vi "Start.vi"(8 "error in (no error)":errorcluster, 10 "Message in":refnum<class "StartMessage.lvclass">, 11 "wavefront sensor in":refnum<class "wavefront sensor.lvclass">) -> (0 "error out":errorcluster, 3 "wavefront sensor out":refnum<class "wavefront sensor.lvclass">)   [LabVIEW 2012, in "wavefront sensor.lvclass"]
doc: "This member function is called when the statemachine in the run.vi receives an 'start' command. It relays the message to all observers of the component.\n\nOverride this member function in your derived class if you need additional start functionality (but don't forget to call the parent method)."
uses:
  wavefront sensor.lvclass
  <vilib>/Distrio/Murmex/StartMessage/StartMessage.lvclass
  <vilib>/Distrio/Murmex/Murmex/Murmex.lvclass
panel:
  # "This member function is called when the statemachine in the run.vi receives an 'start' command. It relays the message to all observers of the component.\n\nOverride this member function in your derived class if you need additional start functionality (but don't forget to call the parent method)."
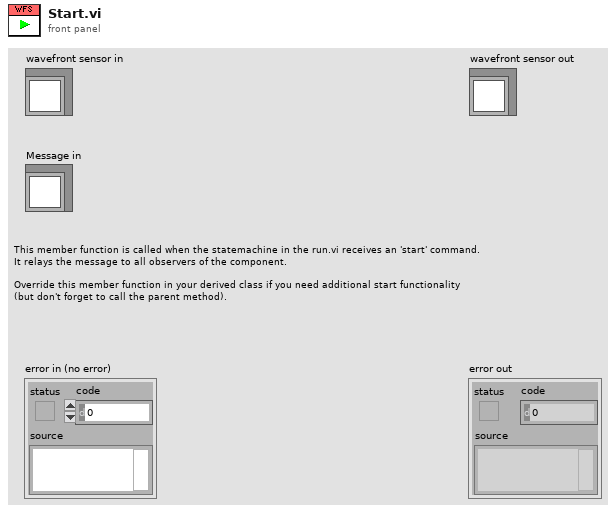
[diagram p1: front panel]
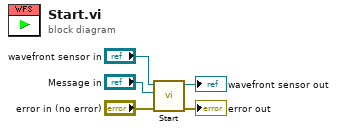
[diagram p0: block diagram]
diagram:
  n1 = call-parent "Start.vi"("error in (no error)"="error in (no error)", "Message in"="Message in", "Murmex in"="wavefront sensor in") -> ("error out"=→"error out":errorcluster, "Murmex out"=→"wavefront sensor out":refnum<class "wavefront sensor.lvclass">)  [unwired: 7 in]
